vi "TDMS_Viewer.vi"   [LabVIEW 2023]
uses:
  <vilib>/Utility/TDMS File Viewer/NI_TDMS File Viewer.lvlib
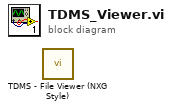
[diagram p0: block diagram]
diagram:
  n1 = call <vilib>:"TDMS - File Viewer (NXG Style).vi"() -> ()  [unwired: 10 in, 2 out]
